vi "Teamprutre Manual Measurement(Bed).vi"(8 "Error In":errorcluster) -> (0 "Error Out":errorcluster)   [LabVIEW 2018]
uses:
  <vilib>/addons/control/pid/pid.llb/PID (DBL).vi
  <vilib>/addons/control/pid/NI_PID_pid.lvlib
panel:
  in  "Duty Cycle\nBed":dbl(slide) scale=0.0..100.0
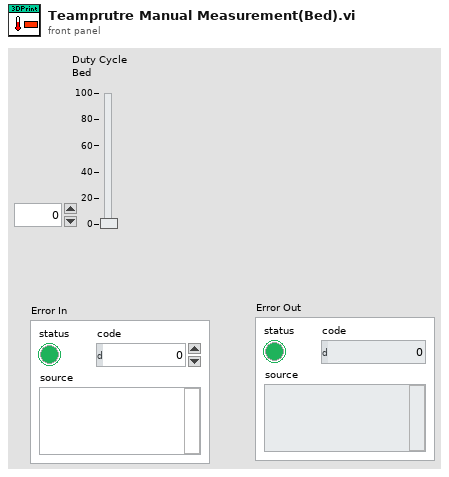
[diagram p1: front panel]
types:
  T1 = cluster{"proportional gain (Kc)":dbl, "integral time (Ti, min)":dbl, "derivative time (Td, min)":dbl}
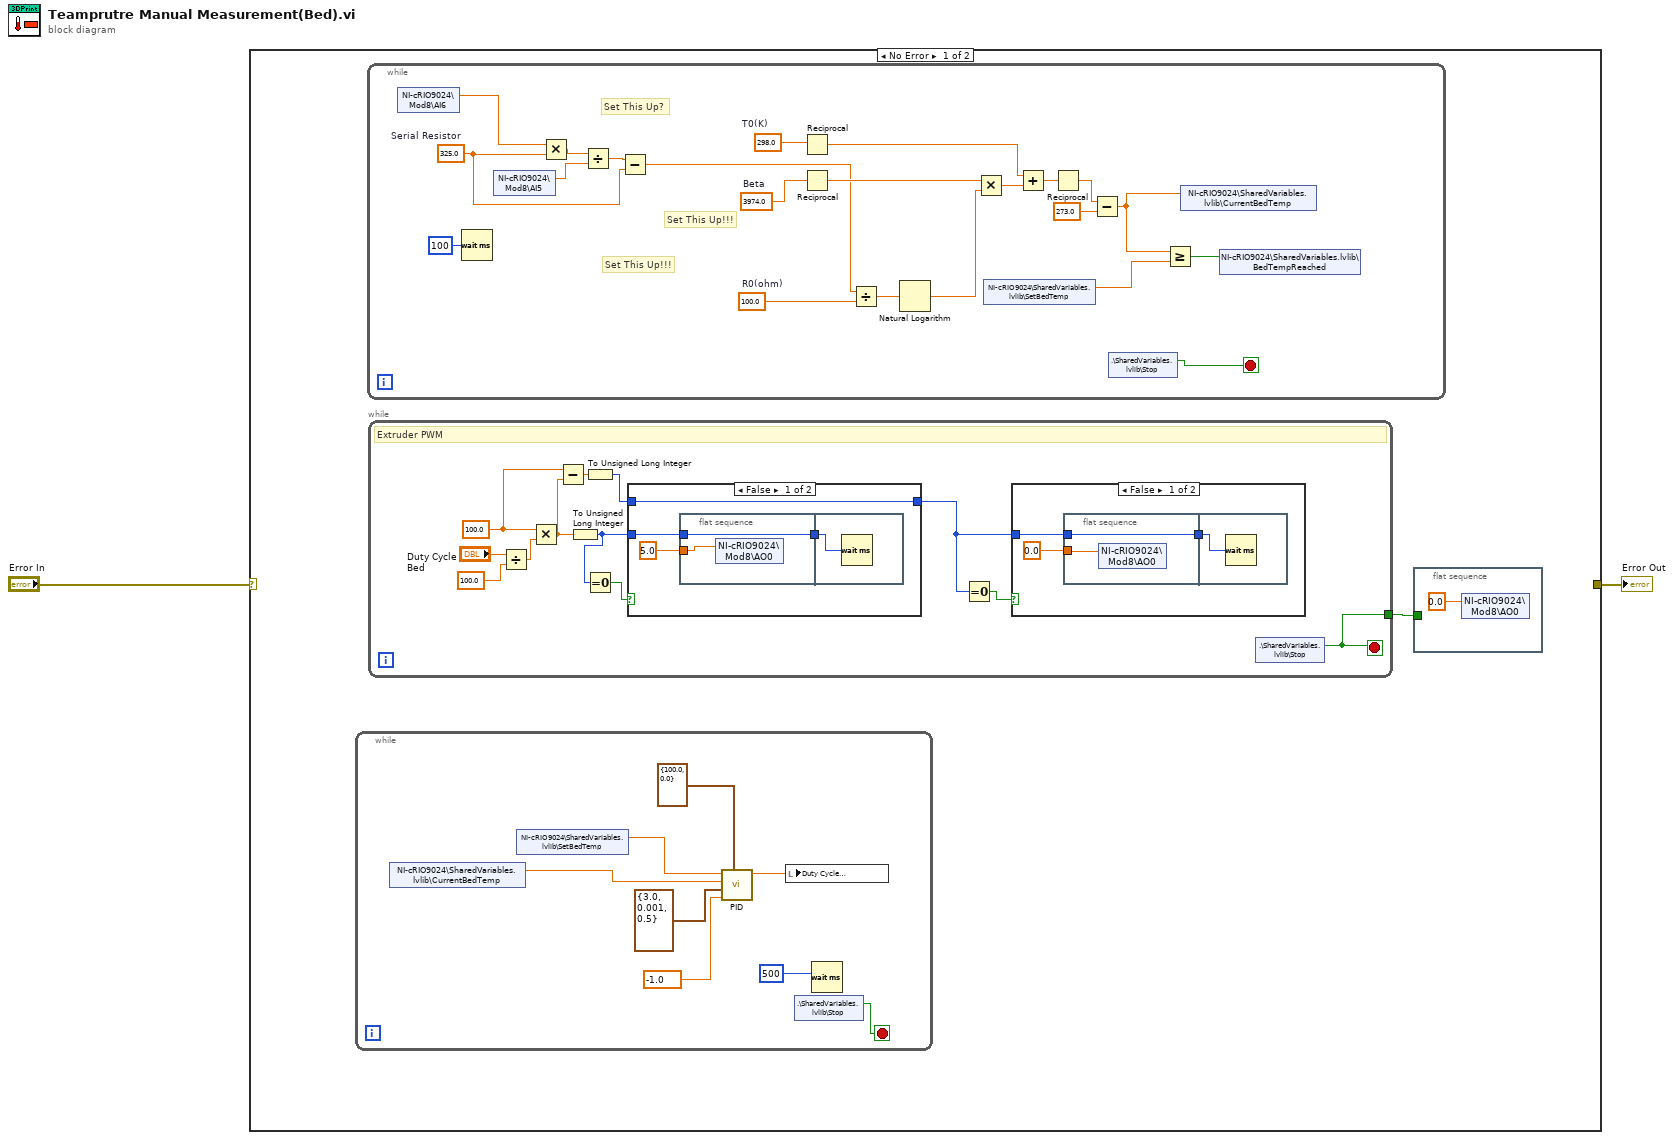
[diagram p0: block diagram]
diagram:
  n1 = case shown="No Error" "Error In" {
    selector: "Error In" -> [_ w61]
    tunnel: [_ w61] -> w1
    frame No Error {
      n2 = while {
        stop <- w11 stop-if-true
        n3 = shared-variable "NI-cRIO9024\\SharedVariables.lvlib\\CurrentBedTemp"() -> (w4:dbl)  [unwired: 1 in, 1 out]
        n4 = shared-variable "NI-cRIO9024\\SharedVariables.lvlib\\SetBedTemp"() -> (w5:dbl)  [unwired: 1 in, 1 out]
        n5 = call-poly <vilib>:"PID.vi"("output range"=cluster{"output high":dbl, "output low":dbl} {"output high"=100.0, "output low"=0.0}, "dt (s)"=-1.0, "PID gains"=T1 {"proportional gain (Kc)"=3.0, "integral time (Ti, min)"=0.001, "derivative time (Td, min)"=0.5}, "process variable"=w4, "setpoint"=w5) -> ("output"=w7:dbl)  [unwired: 5 in, 1 out]
        n6 = local write "Duty Cycle\nBed"(w7) -> ()
        n7 = shared-variable ".\\SharedVariables.lvlib\\Stop"() -> (w11:bool)  [unwired: 1 in, 1 out]
        n8 = Wait (ms)(milliseconds to wait=u32 500 ("PID dt")) -> ()  [unwired: 1 out]
      }
      n9 = while {
        stop <- w59 stop-if-true
        w42 = 325.0  # Serial Resistor
        w58 = 100.0  # R0(ohm)
        w55 = 298.0  # T0(K)
        w56 = 3974.0  # Beta
        # "Set This Up?"
        # "Set This Up!!!"
        # "Set This Up!!!"
        n10 = shared-variable "NI-cRIO9024\\Mod8\\AI6"() -> (w41:dbl)  [unwired: 1 in, 1 out]
        n11 = Wait (ms)(milliseconds to wait=u32 100) -> ()  [unwired: 1 out]
        n12 = shared-variable "NI-cRIO9024\\Mod8\\AI5"() -> (w40:dbl)  [unwired: 1 in, 1 out]
        n13 = Multiply(x=w41, y=w42) -> (x*y=w44:dbl)
        n14 = Divide(x=w44, y=w40) -> (x/y=w43:dbl)
        n15 = Subtract(x=w43, y=w42) -> (x-y=w39:dbl)
        n16 = Reciprocal(x=w55) -> (1/x=w51:dbl)
        n17 = Reciprocal(x=w56) -> (1/x=w54:dbl)
        n18 = Divide(x=w39, y=w58) -> (x/y=w57:dbl)
        n19 = Natural Logarithm(1:w57) -> (0:w53:dbl)
        n20 = Multiply(x=w54, y=w53) -> (x*y=w52:dbl)
        n21 = shared-variable "NI-cRIO9024\\SharedVariables.lvlib\\SetBedTemp"() -> (w47:dbl)  [unwired: 1 in, 1 out]
        n22 = Add(x=w51, y=w52) -> (x+y=w50:dbl)
        n23 = Reciprocal(x=w50) -> (1/x=w49:dbl)
        n24 = Subtract(x=w49, y=273.0) -> (x-y=w45:dbl)
        n25 = shared-variable ".\\SharedVariables.lvlib\\Stop"() -> (w59:bool)  [unwired: 1 in, 1 out]
        n26 = Greater Or Equal?(x=w45, y=w47) -> (x >= y?=w46:bool)
        n27 = shared-variable "NI-cRIO9024\\SharedVariables.lvlib\\CurrentBedTemp"(w45) -> ()  [unwired: 1 in, 1 out]
        n28 = shared-variable "NI-cRIO9024\\SharedVariables.lvlib\\BedTempReached"(w46) -> ()  [unwired: 1 in, 1 out]
      }
      n29 = while {
        tunnel: [w13] -> w3
        stop <- w13 stop-if-true
        w20 = 100.0 ("milliseconds to wait")
        # "Extruder PWM"
        n30 = Divide(x="Duty Cycle\nBed", y=100.0) -> (x/y=w22:dbl)
        n31 = Multiply(x=w20, y=w22) -> (x*y=w21:dbl)
        n32 = Subtract(x=w20, y=w21) -> (x-y=w19:dbl)
        n33 = To Unsigned Long Integer(number=w21) -> (unsigned 32bit integer=w14:u32)
        n34 = To Unsigned Long Integer(number=w19) -> (unsigned 32bit integer=w16:u32)
        n35 = Equal To 0?(x=w14) -> (x = 0?=w18:bool)
        n36 = case shown="False" w18 {
          tunnel: w14 -> [w33 _]
          tunnel: w16 -> [w31 w38]
          tunnel: [w31 w38] -> w15
          frame False {
            n37 = flat-sequence {
              tunnel: [w36] -> w34
              tunnel: w33 -> [w36]
              tunnel: 5.0 ("milliseconds to wait") -> [w35]
              tunnel: w34 -> [w37]
              frame #0 {
                n38 = shared-variable "NI-cRIO9024\\Mod8\\AO0"(w35) -> ()  [unwired: 1 in, 1 out]
              }
              frame #1 {
                n39 = Wait (ms)(milliseconds to wait=w37) -> ()  [unwired: 1 out]
              }
            }
          }
          frame True {
          }
        }
        n40 = Equal To 0?(x=w15) -> (x = 0?=w17:bool)
        n41 = case shown="False" w17 {
          tunnel: w15 -> [w26 _]
          frame False {
            n42 = flat-sequence {
              tunnel: [w29] -> w27
              tunnel: w26 -> [w29]
              tunnel: 0.0 ("milliseconds to wait") -> [w28]
              tunnel: w27 -> [w30]
              frame #0 {
                n43 = shared-variable "NI-cRIO9024\\Mod8\\AO0"(w28) -> ()  [unwired: 1 in, 1 out]
              }
              frame #1 {
                n44 = Wait (ms)(milliseconds to wait=w30) -> ()  [unwired: 1 out]
              }
            }
          }
          frame True {
          }
        }
        n45 = shared-variable ".\\SharedVariables.lvlib\\Stop"() -> (w13:bool)  [unwired: 1 in, 1 out]
      }
      n46 = flat-sequence {
        tunnel: w3 -> [_]
        frame #0 {
          n47 = shared-variable "NI-cRIO9024\\Mod8\\AO0"(0.0 ("AO4")) -> ()  [unwired: 1 in, 1 out]
        }
      }
    }
    frame Error {
    }
  }
  "Error Out" <- w1
